vi "Init Resolve.vi"(11 "Map in":refnum<class "Map.lvclass">) -> (1 "New Map out":refnum<class "Map.lvclass">)   [LabVIEW 2020, in "SquareBattle.lvlib" / "Map.lvclass"]
uses:
  Map.lvclass
  Map.lvclass/Map.ctl
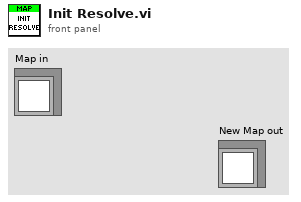
[diagram p1: front panel]
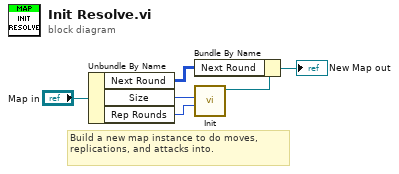
[diagram p0: block diagram]
diagram:
  # "Build a new map instance to do moves, replications, and attacks into."
  n1 = Unbundle By Name("Map in") -> ("Next Round"=w2:u32[][], "Size"=w5:i32, "Rep Rounds"=w4:u32)
  n2 = call "Init.vi"("Replication Rounds"=w4, "Size"=w5) -> ("Map out"=w3:refnum<class "Map.lvclass">)  [unwired: 8 in, 1 out]
  n3 = Bundle By Name(cluster=w3, "Next Round"=w2) -> (→"New Map out":refnum<class "Map.lvclass">)
